vi "DriveModuleOpen.vi"(6 "Magnet Offset (Degrees)":dbl, 7 "ModualNamePrefix":string, 8 "error in":errorcluster, 9 "EncoderCanID":u8, 10 "SpinCanID":u8, 11 "TravelCanID":u8) -> (0 "error out":errorcluster)   [LabVIEW 2023]
uses:
  <vilib>/Rock Robotics/WPI/ThirdParty/REV Robotics/REVLib/Typedef/Spark MAX Idle Mode.ctl
  <vilib>/Rock Robotics/WPI/ThirdParty/REV Robotics/REVLib/SubVI/Public/SPARK Open Brushless.vi
  <vilib>/Rock Robotics/WPI/ThirdParty/REV Robotics/REVLib/SubVI/Public/SPARK Configure Basic Idle Mode.vi
  <vilib>/Rock Robotics/WPI/ThirdParty/REV Robotics/REVLib/SubVI/Public/SPARK Configure Basic Ramp Rate.vi
  <vilib>/Rock Robotics/WPI/ThirdParty/REV Robotics/REVLib/SubVI/Public/SPARK Configure Encoder Conversion Factors.vi
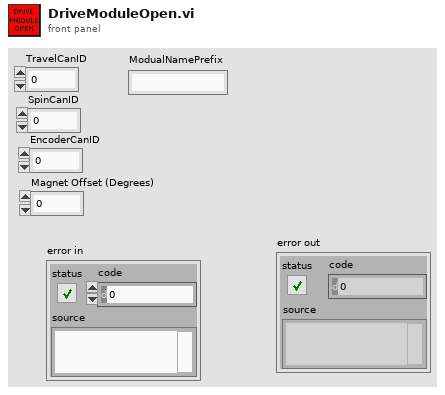
[diagram p1: front panel]
types:
  T1 = typedef "Spark MAX Idle Mode.ctl" = enum16{"Coast", "Brake"}
  T2 = typedef "WPI_MotorControlDeviceRef.ctl" = cluster{"DeviceStatus":errorcluster, "Type":T3, "PWM":cluster{"PWM Channel":T4, "DeadBand":T5}, "CAN":cluster{"Device Number":u8, "SetOutput VI Ref":variant, "GetOutput VI Ref":variant, "Enable VI Ref":variant, "Disable VI Ref":variant, "Data":variant}, "Invert":bool, "DIO PWM":cluster{"PWM \"Enable\" Channel":T4, "DIOChannel":T6, "PWM Rate":dbl}}
  T3 = typedef "WPI_MotorControlType.ctl" = enum16{"PWM", "CAN", "DIO PWM"}
  T4 = typedef "FPGA_DIOPWMChannel.ctl" = enum8{"PWM 0", "PWM 1", "PWM 2", "PWM 3", "PWM 4", "PWM 5", "PWM 6", "PWM 7", "PWM 8", "PWM 9", "PWM MXP 0", "PWM MXP 1", "PWM MXP 2", "PWM MXP 3", "PWM MXP 4", "PWM MXP 5", "PWM MXP 6", "PWM MXP 7", "PWM MXP 8", "PWM MXP 9", "Invalid"}
  T5 = typedef "WPI_PWMDeadband.ctl" = cluster{"Name":string, "maxPositivePwm":i32, "minPositivePwm":i32, "centerPwm":i32, "maxNegativePwm":i32, "minNegativePwm":i32, "angularRange":u16}
  T6 = typedef "FPGA_DIOChannel.ctl" = enum8{"DIO 0", "DIO 1", "DIO 2", "DIO 3", "DIO 4", "DIO 5", "DIO 6", "DIO 7", "DIO 8", "DIO 9", "DIO MXP 0", "DIO MXP 1", "DIO MXP 2", "DIO MXP 3", "DIO MXP 4", "DIO MXP 5", "DIO MXP 6", "DIO MXP 7", "DIO MXP 8", "DIO MXP 9", "DIO MXP 10", "DIO MXP 11", "DIO MXP 12", "DIO MXP 13", "DIO MXP 14", "DIO MXP 15", "SPI Port CS1", "SPI Port CS2", "SPI Port CS3", "SPI Port MISO", "SPI Port MOSI", "Invalid"}
  T7 = typedef "CTRE_Phoenix_CANcoder_DeviceRef.ctl" = cluster{"DeviceStatus":errorcluster, "Device Number":u8, "Handle":u64, "UsageFrame":u32, "Library Path":path}
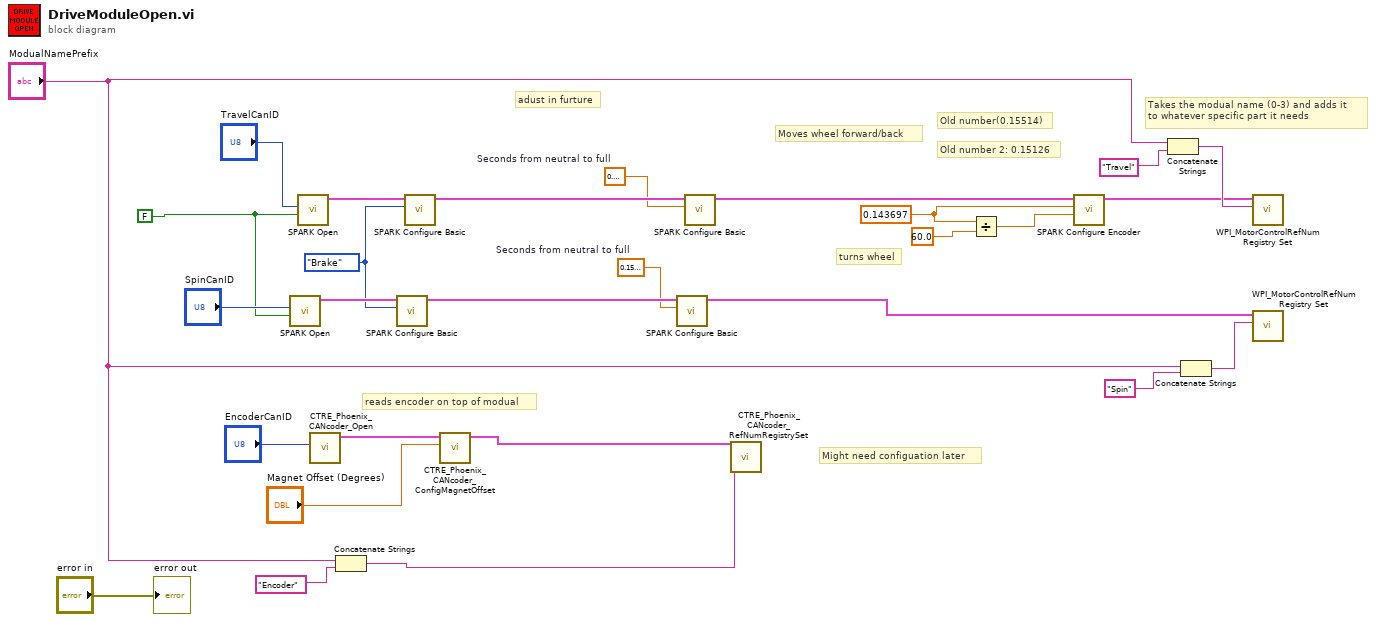
[diagram p0: block diagram]
diagram:
  w1 = sgl 0.15  # Seconds from neutral to full
  w12 = sgl 0.3  # Seconds from neutral to full
  w11 = 0.143697 ("Position Factor (1)")
  w4 = Spark_MAX_Idle_Mode."Brake" ("Idle Mode")
  w6 = FALSE ("Invert")
  # "adust in furture"
  # "Old number 2: 0.15126"
  # "Old number(0.15514)"
  # "reads encoder on top of modual"
  # "turns wheel"
  # "Moves wheel forward/back"
  # "Might need configuation later"
  # "Takes the modual name (0-3) and adds it \nto whatever specific part it needs"
  n1 = call-poly <vilib>:"SPARK Open.vi"("Invert"=w6, "Device Number"="SpinCanID") -> ("MotorControlDeviceRef"=w5:T2)  [unwired: 8 in, 1 out]
  n2 = call-poly <vilib>:"SPARK Open.vi"("Invert"=w6, "Device Number"="TravelCanID") -> ("MotorControlDeviceRef"=w14:T2)  [unwired: 8 in, 1 out]
  n3 = call <vilib>:"CTRE_Phoenix_CANcoder_Open.vi"("Device Number"="EncoderCanID") -> ("CTRE_CANcoder_DeviceRef"=w18:T7)  [unwired: 9 in, 1 out]
  n4 = Concatenate Strings("ModualNamePrefix", "Encoder" ("refnum name")) -> (w21:string)
  n5 = call-poly <vilib>:"SPARK Configure Basic.vi"("Idle Mode"=w4, "MotorControlDeviceRef in"=w5) -> ("MotorControlDeviceRef out"=w3:T2)  [unwired: 8 in, 1 out]
  n6 = call-poly <vilib>:"SPARK Configure Basic.vi"("Idle Mode"=w4, "MotorControlDeviceRef in"=w14) -> ("MotorControlDeviceRef out"=w13:T2)  [unwired: 8 in, 1 out]
  n7 = call <vilib>:"CTRE_Phoenix_CANcoder_ConfigMagnetOffset.vi"("Magnet Offset (Degrees)"="Magnet Offset (Degrees)", "CTRE_CANcoder_DeviceRef"=w18) -> ("CTRE_CANcoder_DeviceRef"=w17:T7)  [unwired: 8 in, 1 out]
  n8 = call-poly <vilib>:"SPARK Configure Basic.vi"("Seconds from neutral to full (0)"=w1, "MotorControlDeviceRef in"=w3) -> ("MotorControlDeviceRef"=w2:T2)  [unwired: 8 in, 1 out]
  n9 = call-poly <vilib>:"SPARK Configure Basic.vi"("Seconds from neutral to full (0)"=w12, "MotorControlDeviceRef in"=w13) -> ("MotorControlDeviceRef"=w9:T2)  [unwired: 8 in, 1 out]
  n10 = call <vilib>:"CTRE_Phoenix_CANcoder_RefNumRegistrySet.vi"("refnum name"=w21, "CTRE_CANcoder_DeviceRef"=w17) -> ()  [unwired: 8 in, 2 out]
  n11 = Divide(x=w11, y=60.0) -> (x/y=w10:dbl)
  n12 = call-poly <vilib>:"SPARK Configure Encoder.vi"("Velocity Conversion Factor"=w10, "Position Conversion Factor"=w11, "MotorControlDeviceRef in"=w9) -> ("MotorControlDeviceRef out"=w8:T2)  [unwired: 7 in, 1 out]
  n13 = Concatenate Strings("ModualNamePrefix", "Travel" ("refnum name")) -> (w27:string)
  n14 = Concatenate Strings("ModualNamePrefix", "Spin" ("refnum name")) -> (w25:string)
  n15 = call <vilib>:"WPI_MotorControlRefNum Registry Set.vi"("refnum name"=w27, "MotorControlDevRef"=w8) -> ()  [unwired: 8 in, 2 out]
  n16 = call <vilib>:"WPI_MotorControlRefNum Registry Set.vi"("refnum name"=w25, "MotorControlDevRef"=w2) -> ()  [unwired: 8 in, 2 out]
  "error out" <- "error in"
